vi "SavedSettingsAppsAndVIs.vi"(8 "error in (no error)":errorcluster, 10 "Tag":string, 11 "SavedSettings in":refnum<vi>) -> (0 "error out":errorcluster, 1 "VIs":map{string, string}(c390), 2 "Apps":map{string, string}(c390), 3 "SavedSettings out":refnum<vi>)   [LabVIEW 2020]
uses:
  <vilib>/regexp/Match Regular Expression.xnode
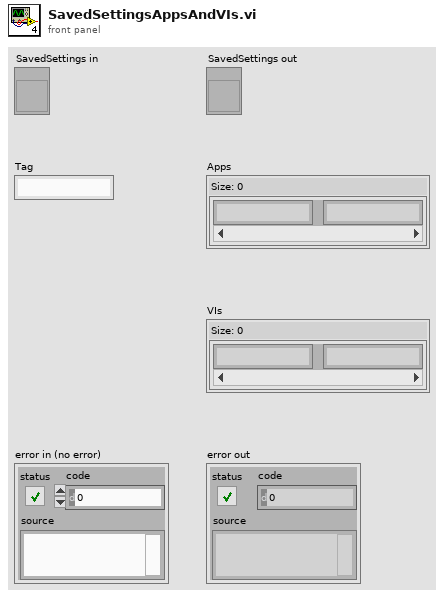
[diagram p1: front panel]
types:
  T1 = cluster{"[0]":map{string, string}, "[1]":map{string, string}}
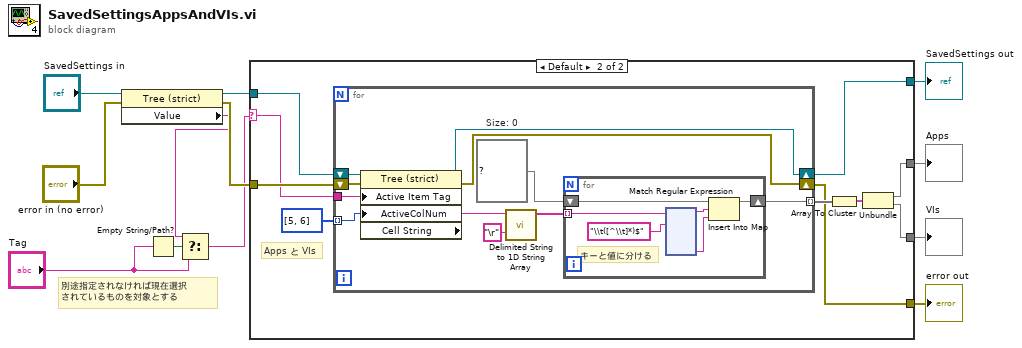
[diagram p0: block diagram]
diagram:
  # "別途指定されなければ現在選択\nされているものを対象とする"
  n1 = property class="Tree (strict)"(reference="SavedSettings in", error in="error in (no error)") -> (reference out=w7:refnum<vi>, error out=w5:errorcluster, "Value"=w2:string)
  n2 = Empty String/Path?(string/path="Tag") -> (empty?=w4:bool)
  n3 = Select(t=w2, s=w4, f="Tag") -> (s? t:f=w1:string)
  n4 = case shown="Default" w1 {
    selector: w1 -> [_ w15]
    tunnel: w7 -> [w13 w24]
    tunnel: [_ w20] -> w11
    tunnel: [_ w19] -> w10
    tunnel: w5 -> [w14 w18]
    tunnel: [w13 w17] -> w9
    tunnel: [w14 w16] -> w8
    frame "" {
    }
    frame Default {
      # "Apps と VIs"
      n5 = for {
        tunnel: i32[] [5, 6] -> [w26] mode=indexing
        tunnel: [w30] -> w22 mode=indexing
        shift-right: [w28] -> w17
        shift-left: w24 -> [w35]
        shift-right: [w29] -> w16
        shift-left: w18 -> [w27]
        tunnel: w15 -> [w25]
        w33 = map{string, string} {}  # Size: 0
        n6 = property class="Tree (strict)"(reference=w35, error in=w27, "Active Item Tag"=w25, "ActiveColNum"=w26) -> (reference out=w28:refnum<vi>, error out=w29:errorcluster, "Cell String"=w31:string)
        n7 = call <vilib>:"Delimited String to 1D String Array.vi"("delimiter"="\r", "delimited string"=w31) -> ("string array"=w34:string[])  [unwired: 9 in]
        n8 = for {
          tunnel: w34 -> [w41] mode=indexing
          shift-right: [w36] -> w30
          shift-left: w33 -> [w39]
          # "キーと値に分ける"
          n9 = xnode "Match Regular Expression"("input string"=w41, "regular expression"="\\t([^\\t]*)$") -> ("before match"=w38:string, "submatch 1"=w37:string)  [unwired: 4 in, 4 out]
          n10 = Insert Into Map(map in=w39, key=w38, value=w37) -> (map out=w36:map{string, string})  [unwired: 2 out]
        }
      }
      n11 = Array To Cluster(array=w22) -> (cluster=w21:T1)
      n12 = Unbundle(w21) -> ("[0]"=w20:map{string, string}, "[1]"=w19:map{string, string})
    }
  }
  "Apps" <- w11
  "VIs" <- w10
  "SavedSettings out" <- w9
  "error out" <- w8
